vi "Set Channel Names.vi"(0 "Display State In":T1, 5 "Names":string[](array[string]), 7 "Validate":bool, 9 "Container State":T2, 11 "error in (no error)":errorcluster) -> (4 "Display State Out":T1, 15 "error out":errorcluster)   [LabVIEW 2020, in "Multichannel (Full).xctl"]
uses:
  Multichannel (Full).xctl
  <vilib>/_xctls/Container State.ctl
  State.ctl
  <vilib>/_xctls/XControlSupport.lvlib
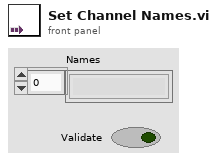
[diagram p1: front panel]
types:
  T1 = typedef "Multichannel (Full).xctl/State.ctl" = cluster{"names":string[], "Reinit?":bool, "Advanced?":bool, "Validate?":bool, "Show persist":bool}
  T2 = typedef "XControlSupport.lvlib/Container State.ctl" = cluster{"Indicator?":bool, "Run Mode?":bool, " Refnum":refnum<vi>}
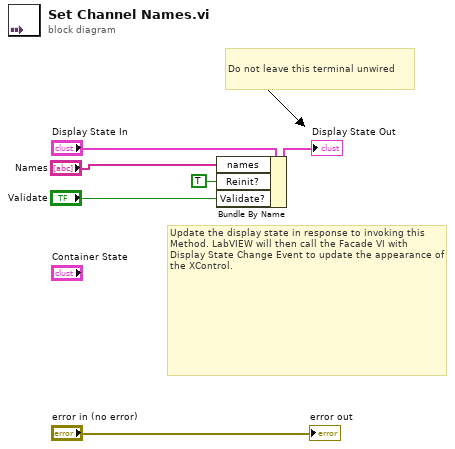
[diagram p0: block diagram]
diagram:
  # "Do not leave this terminal unwired"
  # "Update the display state in response to invoking this Method. LabVIEW will then call the Facade VI with Display State Change Event to update the appearance of the XControl."
  n1 = Bundle By Name(cluster="Display State In", "names"="Names", "Reinit?"=TRUE, "Validate?"="Validate") -> (→"Display State Out":T1)
  "error out" <- "error in (no error)"
